vi "run.vi"(8 "error in (no error)":errorcluster, 11 "Stimulator090724Scaffold in":refnum<class "Stimulator090724Scaffold.lvclass">) -> (0 "error out":errorcluster, 3 "Stimulator090724Scaffold out":refnum<class "Stimulator090724Scaffold.lvclass">)   [LabVIEW 2010, in "Stimulator090724Scaffold.lvclass"]
uses:
  Stimulator090724Scaffold.lvclass
  common/classes/GenericToplevelComponent/GenericToplevelComponent/common_trigger_enum.ctl
  GenericStimulator/GenericStimulator/GenericStimulator.lvclass
  common/classes/GenericComponent/GenericComponent/class_data.vi
  common/classes/GenericToplevelComponent/GenericToplevelComponent/GenericToplevelComponent.lvclass
  common/classes/GenericComponent/GenericComponent/GenericComponent.lvclass
panel:
  out "statechart error":errorcluster
  out "statechart loop counter":i32
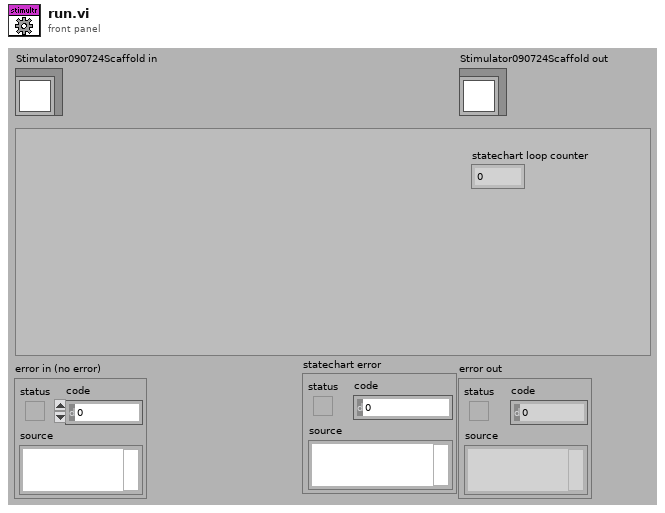
[diagram p1: front panel]
types:
  T1 = typedef "GenericToplevelComponent.lvclass/common_trigger_enum.ctl" = enum16{"NULL", "initialise", "terminate", "fetch command", "fetch data", "attach observer", "register as observer", "detach observer", "acknowledge", "start", "stop", "sweep started", "sweep finished", "experiment started", "experiment stopped"}
  T2 = typedef "Stimulator090724Scaffold.lvclass/internal_trigger_enum.ctl" = enum16{"NULL", "initialise", "terminate", "start sweep", "stop sweep", "start continuous stimulation", "stop continuous stimulation"}
  T3 = typedef "main_trigger_enum.ctl" = enum16{"NULL", "initialise", "terminate", "start", "stop", "change objective", "change experimentController", "change imagingMode", "save notebook", "started saving", "finished saving", "expCtr ready", "expCtr missing", "imgMd ready", "imgMd missing", "scanHd ready", "scanHd missing", "DAQ ready", "DAQ missing", "imgAsm ready", "imgAsm missing", "dataColl ready", "dataColl missing", "display ready", "display missing", "analysr ready", "analysr missing", "instrmnt ready", "instrmnt missing", "stimltr ready", "stimltr missing", "stage ready", "stage missing"}
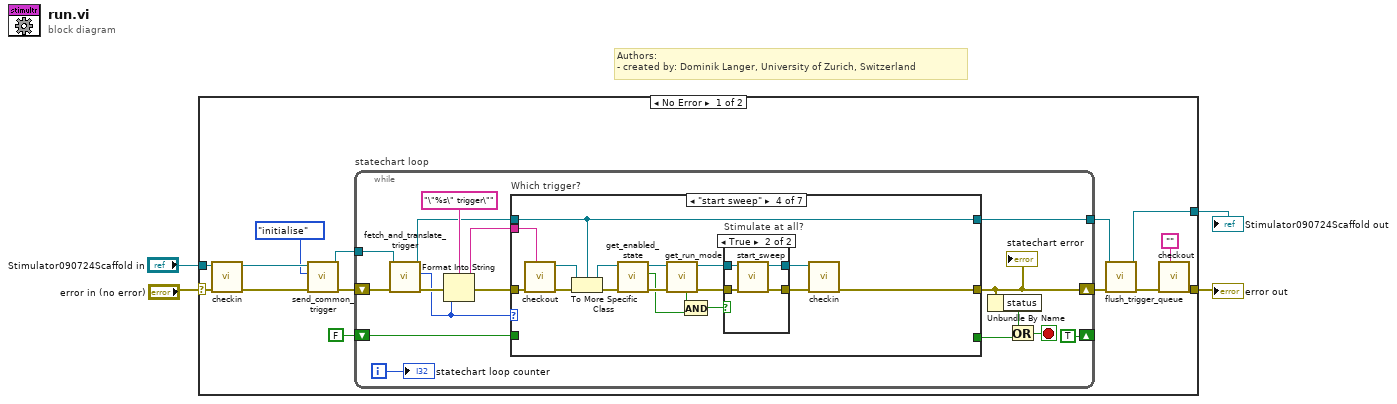
[diagram p0: block diagram]
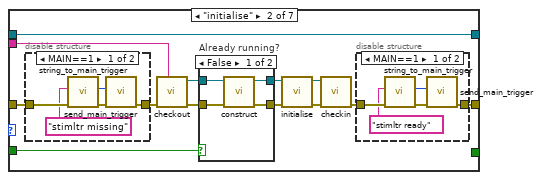
[diagram p3: hidden frame]
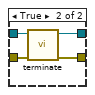
[diagram p6: hidden frame]
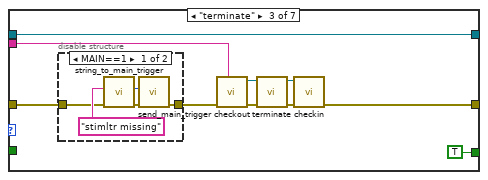
[diagram p7: hidden frame]
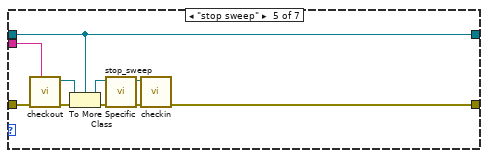
[diagram p10: hidden frame]
diagram:
  # "Authors: \n- created by: Dominik Langer, University of Zurich, Switzerland"
  n1 = case shown="No Error" "error in (no error)" {
    selector: "error in (no error)" -> [w12 w124]
    tunnel: "Stimulator090724Scaffold in" -> [w11 w123]
    tunnel: [w17 w124] -> w2
    tunnel: [w13 w123] -> w1
    frame No Error {
      n2 = call-dynamic "checkin.vi"("error in (no error)"=w12, "GenericStimulator in"=w11) -> ("error out"=w10:errorcluster, "GenericStimulator out"=w8:refnum<class "Stimulator090724Scaffold.lvclass">)  [unwired: 8 in]
      n3 = call-dynamic "send_common_trigger.vi"("error in (no error)"=w10, "trigger"=common_trigger_enum."initialise", "GenericToplevelComponent in"=w8) -> ("error out"=w9:errorcluster, "GenericToplevelComponent out"=w7:refnum<class "Stimulator090724Scaffold.lvclass">)  [unwired: 6 in, 1 out]
      n4 = while "statechart loop" {
        shift-right: [w23] -> w15
        shift-left: w9 -> [w32]
        shift-right: [TRUE] -> _
        shift-left: FALSE -> [w20]
        tunnel: w7 -> [w31]
        tunnel: [w19] -> w6
        i -> [w33]
        stop <- w30 stop-if-true
        n5 = call-dynamic "fetch_and_translate_trigger.vi"("error in (no error)"=w32, "Stimulator090724Scaffold in"=w31) -> ("error out"=w29:errorcluster, "statechart trigger"=w26:T2, "Stimulator090724Scaffold out"=w24:refnum<class "Stimulator090724Scaffold.lvclass">)  [unwired: 6 in, 1 out]
        n6 = Format Into String(format string="\"%s\" trigger\"", error in=w29, w26) -> (resulting string=w25:string, error out=w28:errorcluster)  [unwired: 1 in]
        n7 = case "Which trigger?" shown="\"start sweep\"" w26 {
          tunnel: w28 -> [w36 w40 w70 w98 w112 w120 w122]
          tunnel: w25 -> [_ w43 w75 w97 w111 _ _]
          tunnel: [w36 w41 w74 w95 w109 w120 w122] -> w23
          tunnel: w24 -> [w35 w37 w72 w96 w110 w119 w121]
          tunnel: [_ _ TRUE _ _ _ _] -> w22
          tunnel: w20 -> [_ w38 _ _ _ _ _]
          tunnel: [w35 w37 w72 w96 w110 w119 w121] -> w19
          frame "NULL", Default {
          }
          frame "initialise" {
            n8 = disable-structure shown="MAIN==1" {
              disable-tunnel: w40 -> [w53 w55]
              disable-tunnel: [w54 w55] -> w39
              frame condition #0 (active) {
                n9 = call "string_to_main_trigger.vi"("error in (no error)"=w53, "trigger string"="stimltr missing") -> ("error out"=w51:errorcluster, "main trigger"=w52:T3)  [unwired: 8 in]
                n10 = call "send_main_trigger.vi"("error in (no error)"=w51, "trigger"=w52) -> ("error out"=w54:errorcluster)  [unwired: 9 in]
              }
              frame condition #1 {
              }
            }
            n11 = call "checkout.vi"("locked by?"=w43, "error in (no error)"=w39) -> ("error out"=w44:errorcluster, "GenericStimulator out"=w49:refnum<class "GenericStimulator.lvclass">)  [unwired: 8 out]
            n12 = case "Already running?" shown="False" w38 {
              tunnel: w44 -> [w65 w69]
              tunnel: [w64 w67] -> w45
              tunnel: [w63 w66] -> w47
              tunnel: w49 -> [w62 w68]
              frame False {
                n13 = call-dynamic "construct.vi"("error in (no error)"=w65, "GenericPlugin in"=w62) -> ("error out"=w63:errorcluster, "GenericPlugin out"=w64:refnum<class "GenericStimulator.lvclass">)  [unwired: 2 in, 6 out]
              }
              frame True {
                n14 = call-dynamic "terminate.vi"("error in (no error)"=w69, "GenericPlugin in"=w68) -> ("error out"=w66:errorcluster, "GenericPlugin out"=w67:refnum<class "GenericStimulator.lvclass">)  [unwired: 8 out]
              }
            }
            n15 = call-dynamic "initialise.vi"("error in (no error)"=w47, "GenericPlugin in"=w45) -> ("error out"=w48:errorcluster, "GenericPlugin out"=w46:refnum<class "GenericStimulator.lvclass">)  [unwired: 8 out]
            n16 = call-dynamic "checkin.vi"("error in (no error)"=w48, "GenericStimulator in"=w46) -> ("error out"=w42:errorcluster)  [unwired: 8 in, 1 out]
            n17 = disable-structure shown="MAIN==1" {
              disable-tunnel: w42 -> [w59 w61]
              disable-tunnel: [w60 w61] -> w41
              frame condition #0 (active) {
                n18 = call "string_to_main_trigger.vi"("error in (no error)"=w59, "trigger string"="stimltr ready") -> ("error out"=w58:errorcluster, "main trigger"=w57:T3)  [unwired: 8 in]
                n19 = call "send_main_trigger.vi"("error in (no error)"=w58, "trigger"=w57) -> ("error out"=w60:errorcluster)  [unwired: 9 in]
              }
              frame condition #1 {
              }
            }
          }
          frame "terminate" {
            n20 = disable-structure shown="MAIN==1" {
              disable-tunnel: w70 -> [w80 w85]
              disable-tunnel: [w84 w85] -> w71
              frame condition #0 (active) {
                n21 = call "string_to_main_trigger.vi"("error in (no error)"=w80, "trigger string"="stimltr missing") -> ("error out"=w82:errorcluster, "main trigger"=w83:T3)  [unwired: 8 in]
                n22 = call "send_main_trigger.vi"("error in (no error)"=w82, "trigger"=w83) -> ("error out"=w84:errorcluster)  [unwired: 9 in]
              }
              frame condition #1 {
              }
            }
            n23 = call "checkout.vi"("locked by?"=w75, "error in (no error)"=w71) -> ("error out"=w79:errorcluster, "GenericStimulator out"=w78:refnum<class "GenericStimulator.lvclass">)  [unwired: 8 out]
            n24 = call-dynamic "terminate.vi"("error in (no error)"=w79, "GenericPlugin in"=w78) -> ("error out"=w76:errorcluster, "GenericPlugin out"=w77:refnum<class "GenericStimulator.lvclass">)  [unwired: 8 out]
            n25 = call-dynamic "checkin.vi"("error in (no error)"=w76, "GenericStimulator in"=w77) -> ("error out"=w74:errorcluster)  [unwired: 8 in, 1 out]
          }
          frame "start sweep" {
            n26 = call "checkout.vi"("locked by?"=w97, "error in (no error)"=w98) -> ("error out"=w101:errorcluster, "GenericStimulator out"=w100:refnum<class "GenericStimulator.lvclass">)  [unwired: 8 out]
            n27 = To More Specific Class(target class=w96, reference=w100, error in=w101) -> (specific class reference=w90:refnum<class "Stimulator090724Scaffold.lvclass">, error out=w92:errorcluster)
            n28 = call-dynamic "get_enabled_state.vi"("error in (no error)"=w92, "GenericStimulator in"=w90) -> ("error out"=w93:errorcluster, "stimulator enabled?"=w88:bool, "GenericStimulator out"=w94:refnum<class "Stimulator090724Scaffold.lvclass">)  [unwired: 7 in]
            n29 = call "get_run_mode.vi"("error in (no error)"=w93, "GenericPlugin in"=w94) -> ("error out"=w91:errorcluster, "GenericPlugin out"=w89:refnum<class "Stimulator090724Scaffold.lvclass">, "is NOT free run?"=w87:bool)  [unwired: 5 in, 2 out]
            n30 = And(x=w87, y=w88) -> (x .and. y?=w86:bool)
            n31 = case "Stimulate at all?" shown="True" w86 {
              tunnel: [w104 w108] -> w102
              tunnel: [w103 w107] -> w99
              tunnel: w91 -> [w104 w106]
              tunnel: w89 -> [w103 w105]
              frame False {
              }
              frame True {
                n32 = call-dynamic "start_sweep.vi"("error in (no error)"=w106, "Stimulator090724Scaffold in"=w105) -> ("error out"=w108:errorcluster, "Stimulator090724Scaffold out"=w107:refnum<class "Stimulator090724Scaffold.lvclass">)  [unwired: 8 out]
              }
            }
            n33 = call-dynamic "checkin.vi"("error in (no error)"=w102, "GenericStimulator in"=w99) -> ("error out"=w95:errorcluster)  [unwired: 8 in, 1 out]
          }
          frame "stop sweep" {
            n34 = call "checkout.vi"("locked by?"=w111, "error in (no error)"=w112) -> ("error out"=w118:errorcluster, "GenericStimulator out"=w117:refnum<class "GenericStimulator.lvclass">)  [unwired: 8 out]
            n35 = To More Specific Class(target class=w110, reference=w117, error in=w118) -> (specific class reference=w116:refnum<class "Stimulator090724Scaffold.lvclass">, error out=w115:errorcluster)
            n36 = call-dynamic "stop_sweep.vi"("error in (no error)"=w115, "Stimulator090724Scaffold in"=w116) -> ("error out"=w114:errorcluster, "Stimulator090724Scaffold out"=w113:refnum<class "Stimulator090724Scaffold.lvclass">)  [unwired: 8 out]
            n37 = call-dynamic "checkin.vi"("error in (no error)"=w114, "GenericStimulator in"=w113) -> ("error out"=w109:errorcluster)  [unwired: 8 in, 1 out]
          }
          frame "start continuous stimulation" {
          }
          frame "stop continuous stimulation" {
          }
        }
        "statechart error" <- w23
        n38 = Unbundle By Name(w23) -> ("status"=w21:bool)
        n39 = Or(x=w21, y=w22) -> (x .or. y?=w30:bool)
        "statechart loop counter" <- w33
      }
      n40 = call-dynamic "flush_trigger_queue.vi"("error in (no error)"=w15, "GenericToplevelComponent in"=w6) -> ("error out"=w14:errorcluster, "GenericToplevelComponent out"=w13:refnum<class "Stimulator090724Scaffold.lvclass">)  [unwired: 8 in]
      n41 = call "checkout.vi"("locked by?"="", "error in (no error)"=w14) -> ("error out"=w17:errorcluster)  [unwired: 9 out]
    }
    frame Error {
    }
  }
  "error out" <- w2
  "Stimulator090724Scaffold out" <- w1
